vi "grating_GUI.vi"(4 "error in (no error)":errorcluster, 7 "connection ID":refnum<k5>) -> (0 "error out":errorcluster)   [LabVIEW 2015]
doc: "Use this template to build a PDA VI for Pocket PC 2002 devices or emulators."
panel:
  out "Grating Names":string
  in  "Cancel":bool
  in  "OK":bool
  in  "Grating #":i32(ring) items=["None", "1", "2", "3"]
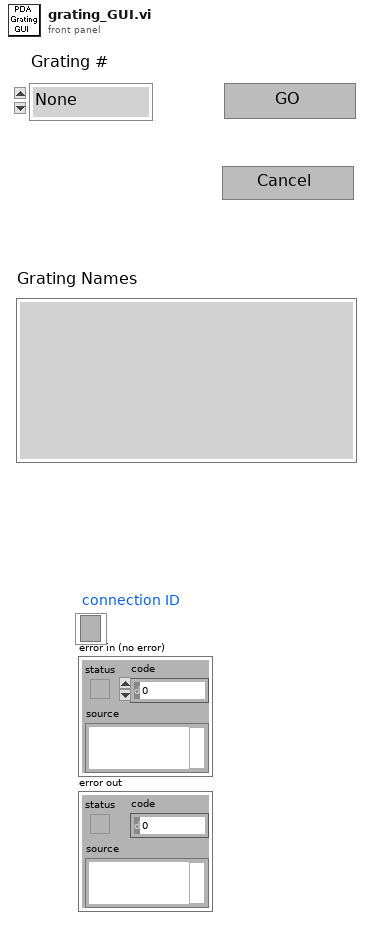
[diagram p1: front panel]
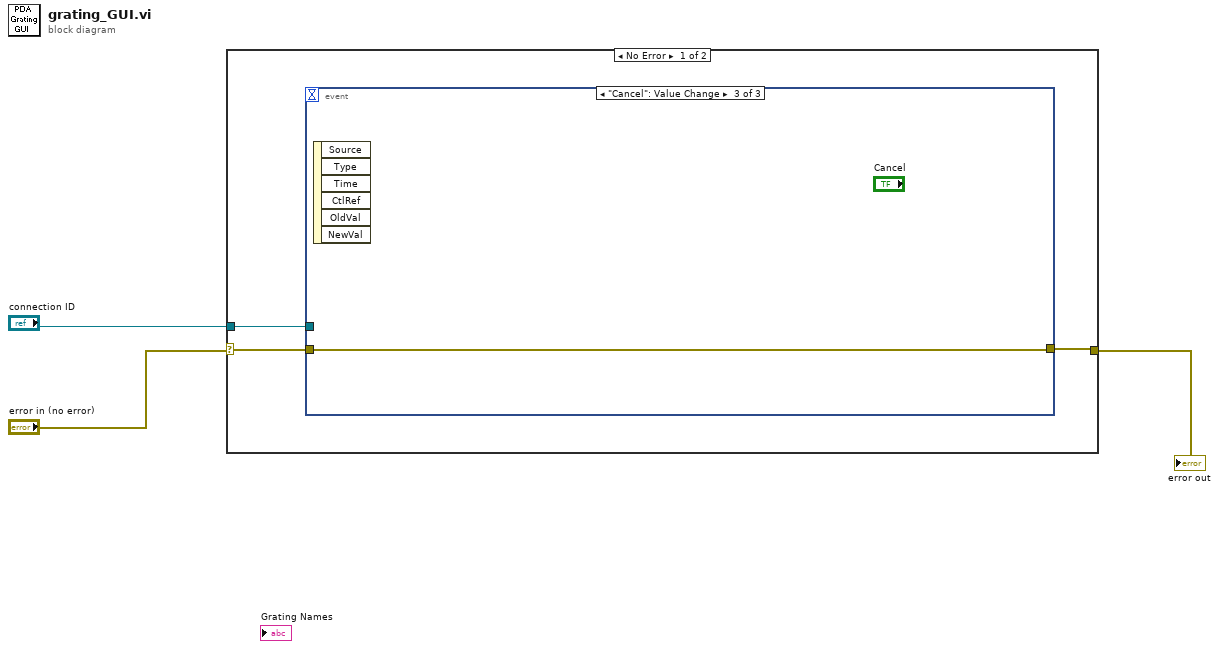
[diagram p0: block diagram]
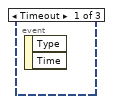
[diagram p2: hidden frame]
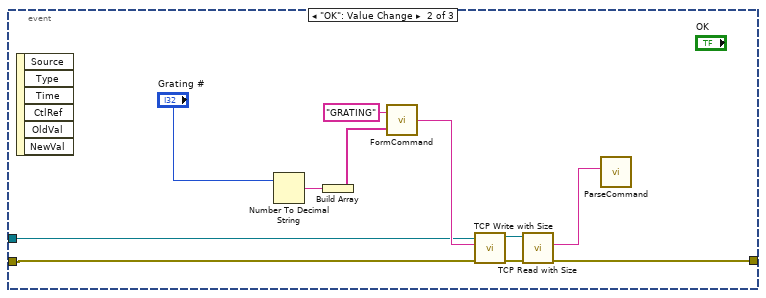
[diagram p3: hidden frame]
diagram:
  n1 = case shown="No Error" "error in (no error)" {
    selector: "error in (no error)" -> [w6 w19]
    tunnel: [w4 w19] -> w3
    tunnel: "connection ID" -> [w5 _]
    frame No Error {
      n2 = event shown="[2] \"Cancel\": Value Change" {
        selector: _ -> [_ _ _]
        dyn-events: _ -> [_ _ _]
        timeout: _ -> [_ _ _]
        tunnel: w6 -> [_ w9 w18]
        tunnel: w5 -> [_ w10 _]
        tunnel: [_ w8 w18] -> w4
        event Timeout {
          n3 = event-data() -> ()  [unwired: 1 in, 2 out]
        }
        event "OK": Value Change {
          n4 = event-data() -> ()  [unwired: 1 in, 6 out]
          n5 = Number To Decimal String(number="Grating #") -> (decimal integer string=w16:string)  [unwired: 1 in]
          n6 = Build Array(w16) -> (w15:string[])
          n7 = call "FormCommand.vi"("Parameters"=w15, "Command"="GRATING") -> ("Command string"=w14:string)
          n8 = call "TCP Write with Size.vi"("error in (no error)"=w9, "data in"=w14, "connection ID"=w10) -> ("error out"=w13:errorcluster, "connection ID out"=w12:refnum<k5>)  [unwired: 6 in, 1 out]
          n9 = call "TCP Read with Size.vi"("error in (no error)"=w13, "connection ID"=w12) -> ("error out"=w8:errorcluster, "data out"=w11:string)  [unwired: 7 in, 1 out]
          n10 = call "ParseCommand.vi"("Command string"=w11) -> ()  [unwired: 2 out]
        }
        event "Cancel": Value Change {
          n11 = event-data() -> ()  [unwired: 1 in, 6 out]
        }
      }
    }
    frame Error {
    }
  }
  "error out" <- w3
